vi "Pass.vi"(0 "Other Array":dbl[](array[numeric]), 1 "Other Boolean Array":bool[](array[boolean]), 2 "Denge Kosulu x2_y2":dbl[][](array[numeric]), 3 "LstBox Refnum":refnum<vi>, 4 "Cluster":T2, 5 "F/P Array Cluster":T1, 6 "Sheet name":string="10k1k", 7 "default values":T3(array[cluster]) {"Kelvin Yk-1" format="%.4p"; "Wagner Yk-1" format="%.4p"; "1R Yk-1" format="%.4p"; "10R Yk-1" format="%.4p"; "Ana Denge Yk-1" format="%.4p"; "Kelvin Yk" format="%.4p"; "Wagner Yk" format="%.4p"; "1R Yk" format="%.4p"; "10R Yk" format="%.4p"; "Ana Denge Yk" format="%.4p"; "Kelvin Xk-1" format="%.4p"; "Wagner Xk-1" format="%.4p"; "1R Xk-1" format="%.4p"; "10R Xk-1" format="%.4p"; "Ana Denge Xk-1" format="%.4p"; "Kelvin Xk" format="%.4p"; "Wagner Xk" format="%.4p"; "1R Xk" format="%.4p"; "10R Xk" format="%.4p"; "Ana Denge Xk" format="%.4p"}, 8 "x1_x2_y1_y2":dbl[][](array[numeric]), 9 "input values":dbl[](array[numeric])) -> (10 "new iterasyon Denge":dbl, 12 "output values":dbl[](array[numeric]), 13 "Output Other Boolean Array":bool[](array[boolean]), 14 "Output Cluster":T2, 15 "Output F/P Array Cluster":T1, 16 "output default values":T3(array[cluster]) {"Kelvin Yk-1" format="%.4p"; "Wagner Yk-1" format="%.4p"; "1R Yk-1" format="%.4p"; "10R Yk-1" format="%.4p"; "Ana Denge Yk-1" format="%.4p"; "Kelvin Yk" format="%.4p"; "Wagner Yk" format="%.4p"; "1R Yk" format="%.4p"; "10R Yk" format="%.4p"; "Ana Denge Yk" format="%.4p"; "Kelvin Xk-1" format="%.4p"; "Wagner Xk-1" format="%.4p"; "1R Xk-1" format="%.4p"; "10R Xk-1" format="%.4p"; "Ana Denge Xk-1" format="%.4p"; "Kelvin Xk" format="%.4p"; "Wagner Xk" format="%.4p"; "1R Xk" format="%.4p"; "10R Xk" format="%.4p"; "Ana Denge Xk" format="%.4p"}, 17 "Output Iterasyon Successful":dbl, 18 "Denge Seçimi":u8=4 min=1 max=5, 19 "end time":string)   [LabVIEW 2014]
uses:
  DB_Global_4_kart-Test.vi
  Sub_VI/show_sensitivity.vi
panel:
  in  "Kelvin F/P Array":dbl[][](array[numeric])
  in  "Wagner F/P Array":dbl[][](array[numeric])
  in  "1R F/P Array":dbl[][](array[numeric])
  in  "10R F/P Array":dbl[][](array[numeric])
  in  "AD F/P Array":dbl[][](array[numeric])
  in  "Frekanslar":dbl[](array[numeric])
  in  "F Values Array":dbl[][](array[numeric])
  in  "extra default values":dbl[][](array[numeric])
  in  "control hz array":dbl[][](array[numeric])
  in  "index r":dbl
  in  "iterasyon Denge":dbl
  in  "change switch":bool
  in  "denge degeri":dbl
  in  "reset values":bool
  in  "ölçüm":u16=3 min=1 max=100
  in  "set":u16=3 min=1 max=100
  in  "frekans index":dbl
  in  "RESET SENS Y":bool
  in  "Iterasyon Successful":dbl
  in  "RESET SENS X":bool
  in  "GPIB In":refnum<visa-resource-name>="GPIB0::8::INSTR"
  in  "pass hz":bool
  out "continue object":bool
  # "Denge Degeri\nIterasyon Successful\nindex r\nolcum\nset\nfrekans index\nIterasyon Denge"
  # "pass hz\nchange switch\nreset values\nreset sens x\nreset sens y"
  # "pass hz\nchange switch\nreset values\nreset sens x\nreset sens y"
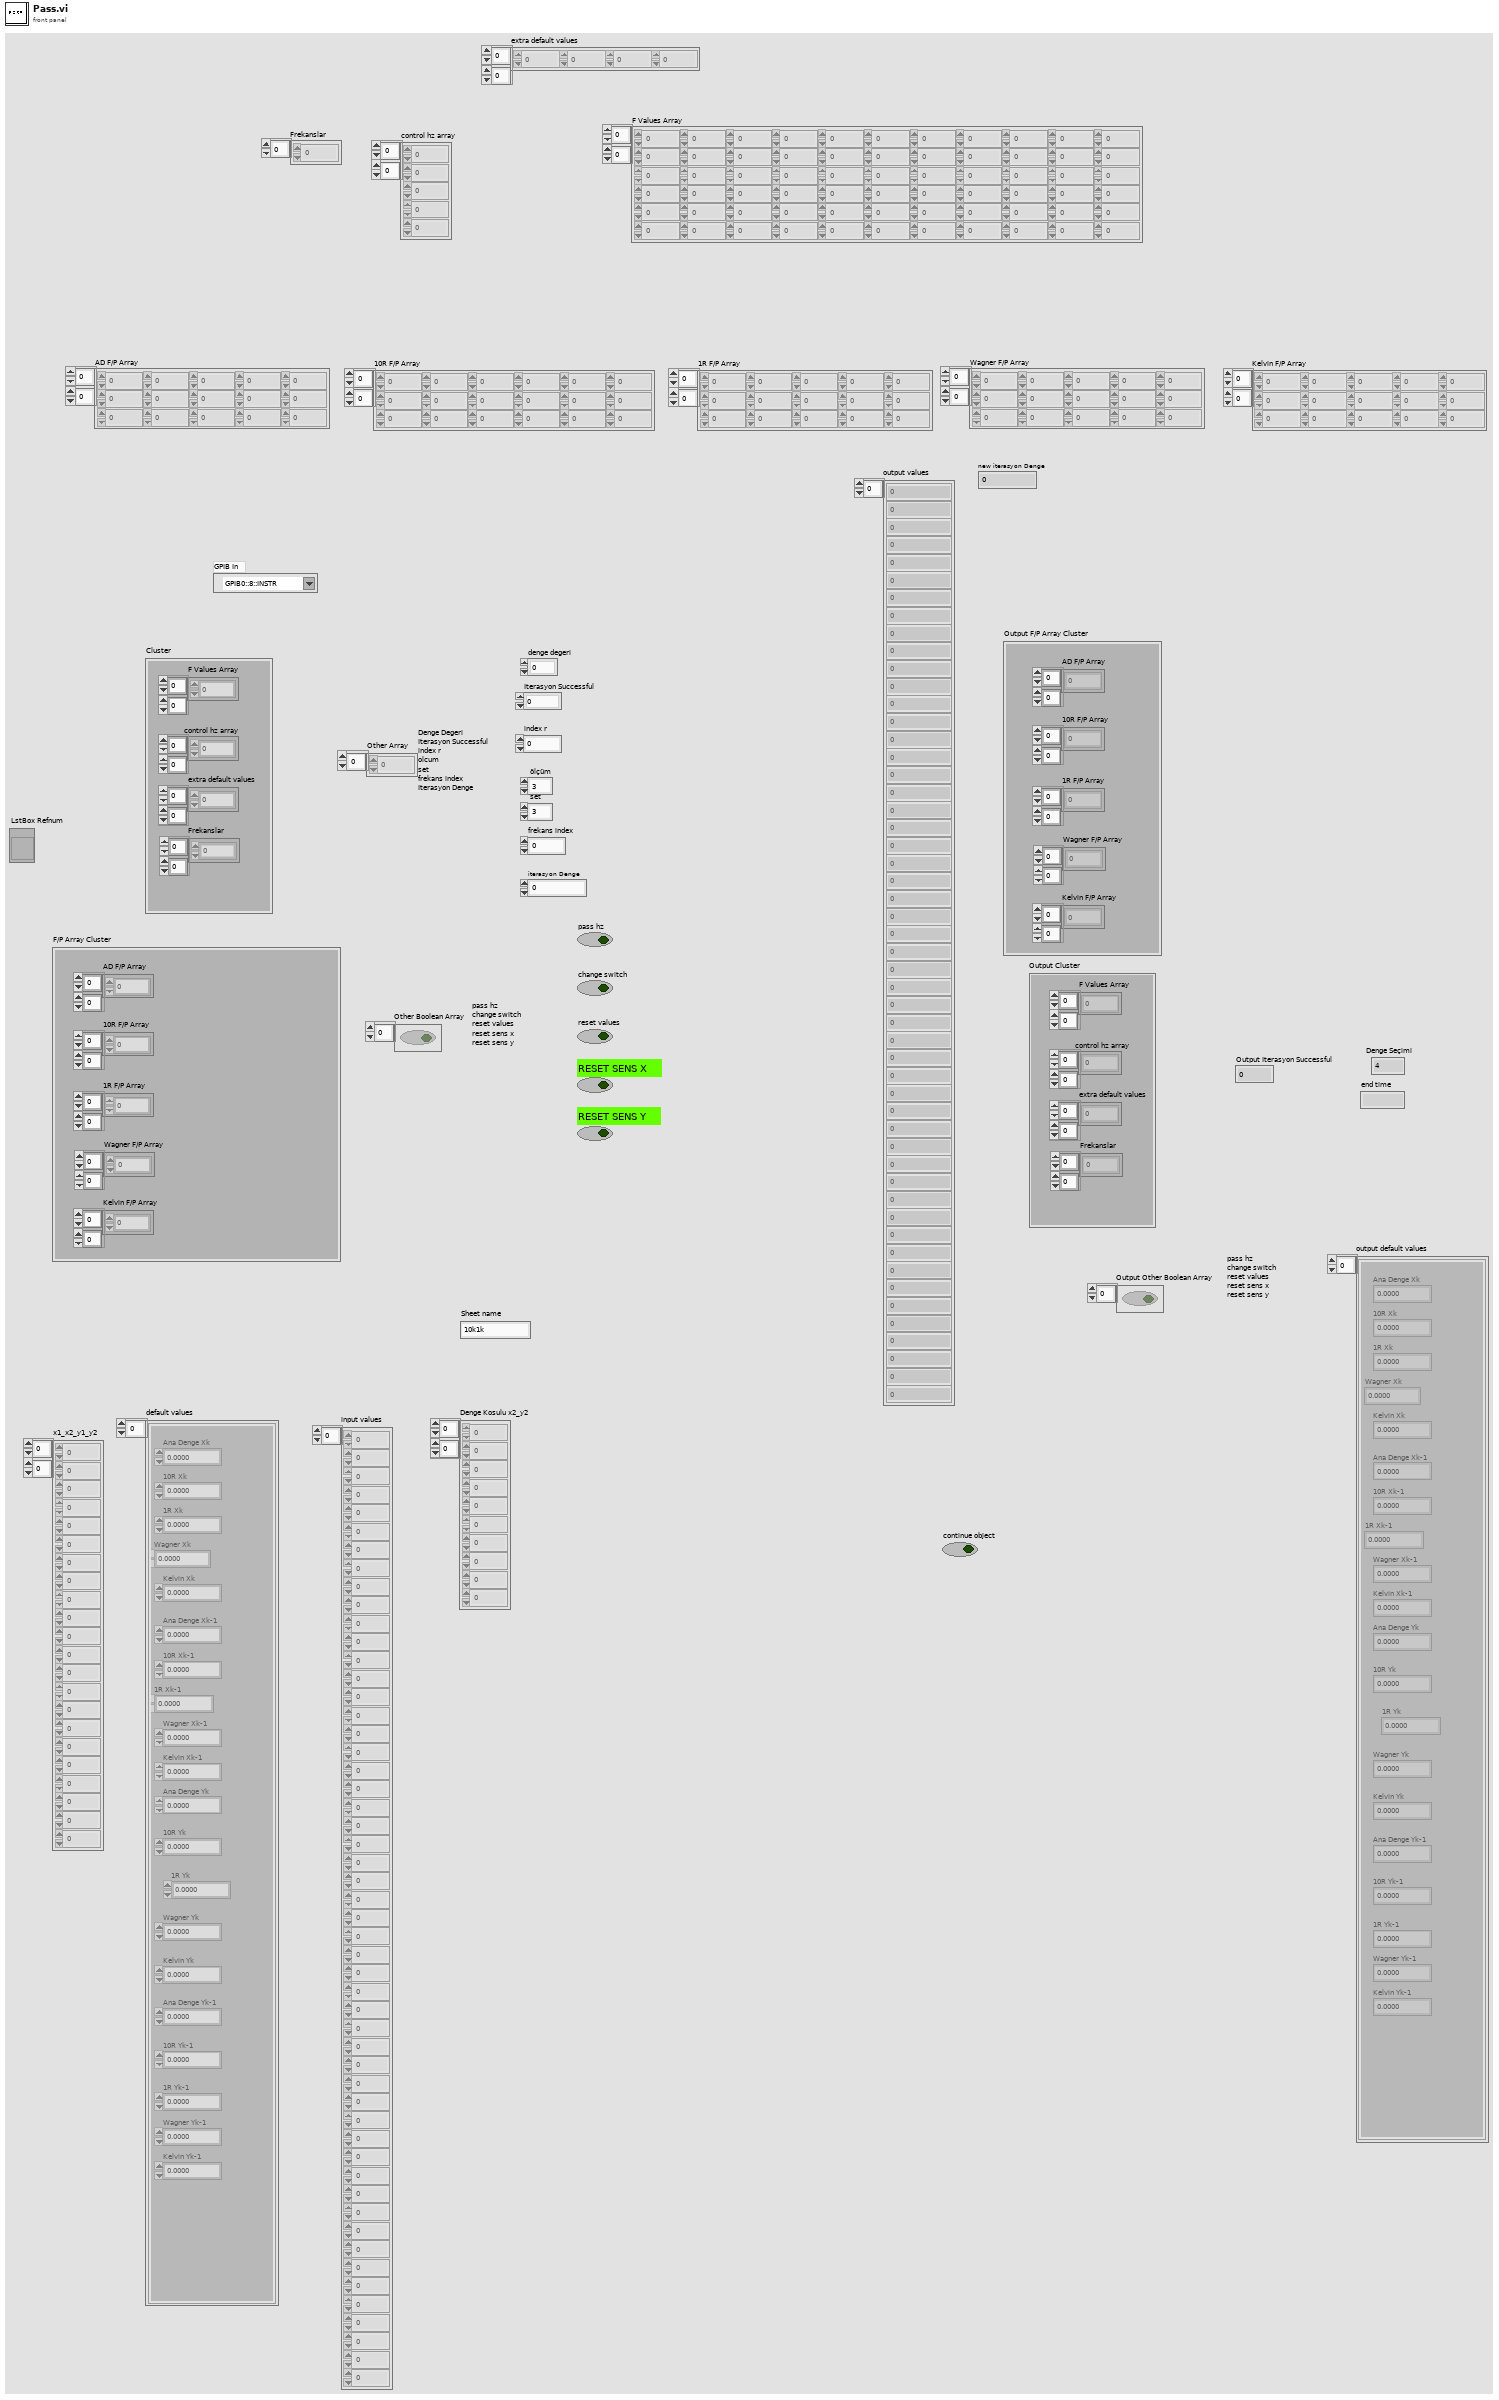
[diagram p1: front panel]
types:
  T1 = cluster{"AD F/P Array":dbl[][], "10R F/P Array":dbl[][], "1R F/P Array":dbl[][], "Wagner F/P Array":dbl[][], "Kelvin F/P Array":dbl[][]}
  T2 = cluster{"F Values Array":dbl[][], "control hz array":dbl[][], "extra default values":dbl[][], "Frekanslar":dbl[][]}
  T3 = cluster{"Ana Denge Xk":dbl, "10R Xk":dbl, "1R Xk":dbl, "Wagner Xk":dbl, "Kelvin Xk":dbl, "Ana Denge Xk-1":dbl, "10R Xk-1":dbl, "1R Xk-1":dbl, "Wagner Xk-1":dbl, "Kelvin Xk-1":dbl, "Ana Denge Yk":dbl, "10R Yk":dbl, "1R Yk":dbl, "Wagner Yk":dbl, "Kelvin Yk":dbl, "Ana Denge Yk-1":dbl, "10R Yk-1":dbl, "1R Yk-1":dbl, "Wagner Yk-1":dbl, "Kelvin Yk-1":dbl}[]
  T4 = cluster{"Ana Denge Xk":dbl, "10R Xk":dbl, "1R Xk":dbl, "Wagner Xk":dbl, "Kelvin Xk":dbl, "Ana Denge Xk-1":dbl, "10R Xk-1":dbl, "1R Xk-1":dbl, "Wagner Xk-1":dbl, "Kelvin Xk-1":dbl, "Ana Denge Yk":dbl, "10R Yk":dbl, "1R Yk":dbl, "Wagner Yk":dbl, "Kelvin Yk":dbl, "Ana Denge Yk-1":dbl, "10R Yk-1":dbl, "1R Yk-1":dbl, "Wagner Yk-1":dbl, "Kelvin Yk-1":dbl}
  T5 = cluster{"[0]":dbl, "[1]":dbl, "[2]":dbl, "[3]":dbl, "[4]":dbl, "[5]":dbl, "[6]":dbl, "[7]":dbl, "[8]":dbl, "[9]":dbl, "[10]":dbl, "[11]":dbl, "[12]":dbl, "[13]":dbl, "[14]":dbl, "[15]":dbl, "[16]":dbl, "[17]":dbl, "[18]":dbl, "[19]":dbl}
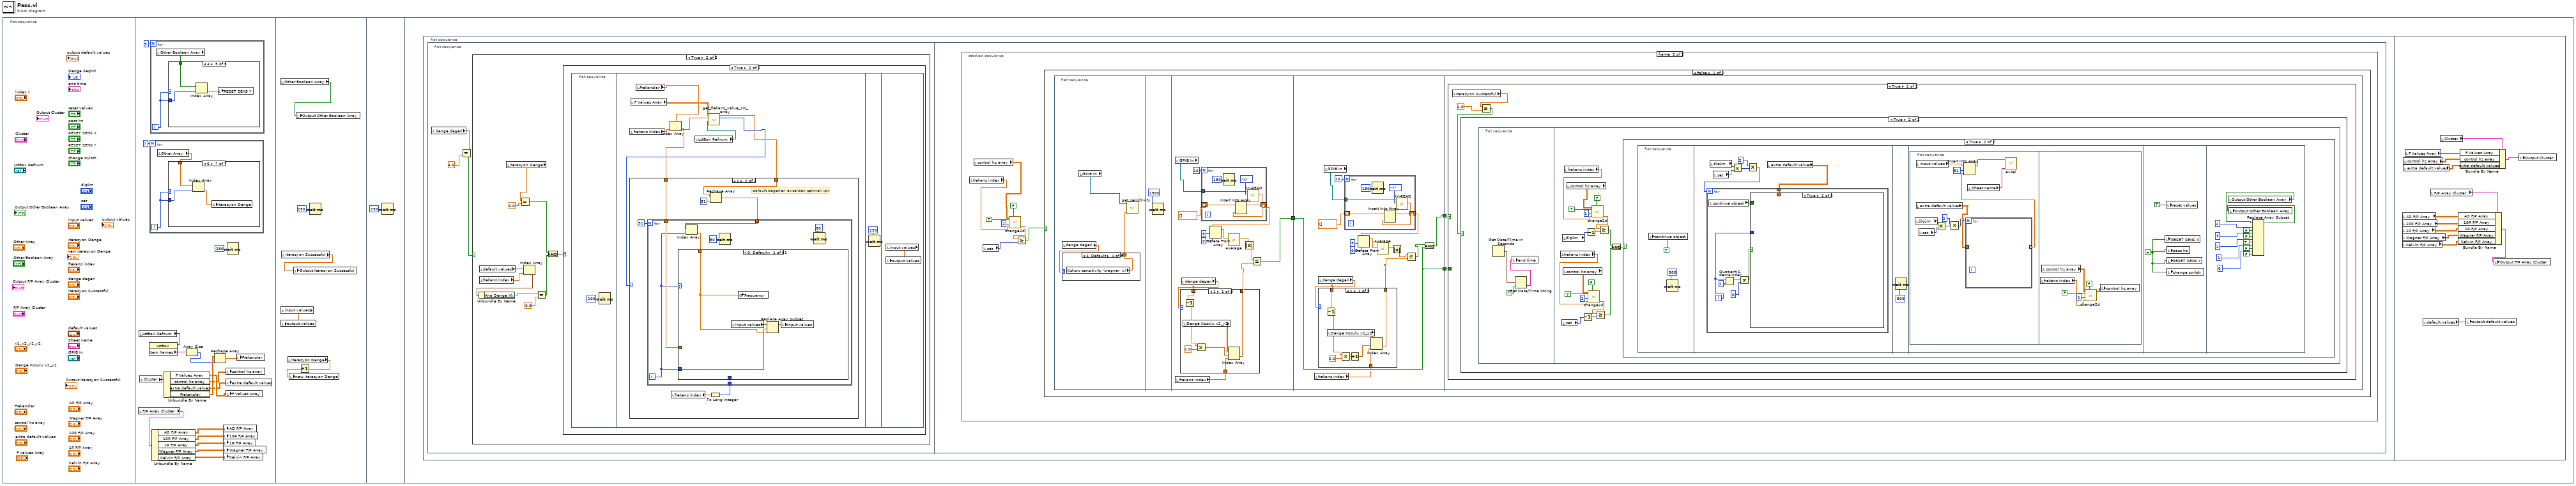
[diagram p0: block diagram]
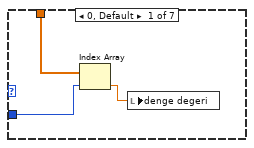
[diagram p2: hidden frame]
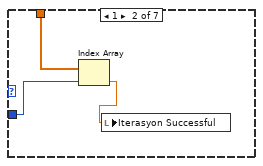
[diagram p3: hidden frame]
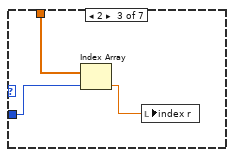
[diagram p4: hidden frame]
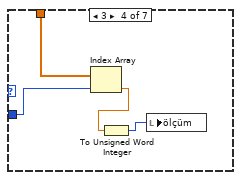
[diagram p5: hidden frame]
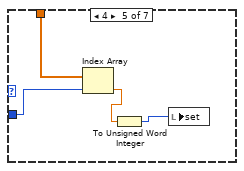
[diagram p6: hidden frame]
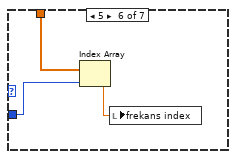
[diagram p7: hidden frame]
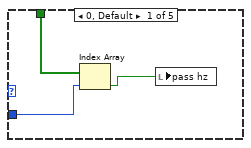
[diagram p8: hidden frame]
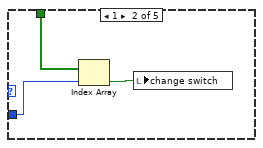
[diagram p9: hidden frame]
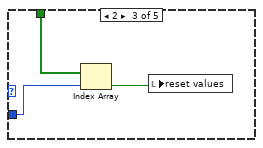
[diagram p10: hidden frame]
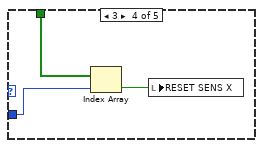
[diagram p11: hidden frame]
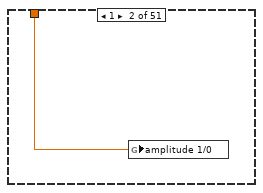
[diagram p15: hidden frame]
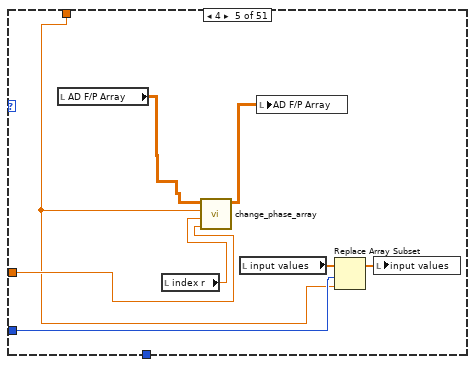
[diagram p18: hidden frame]
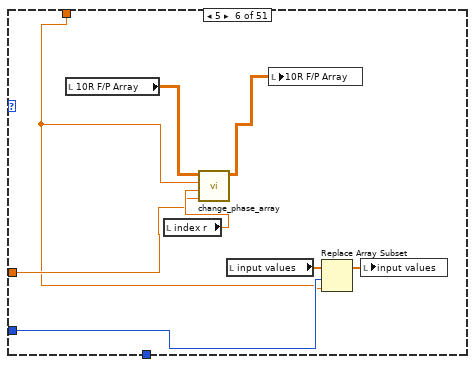
[diagram p19: hidden frame]
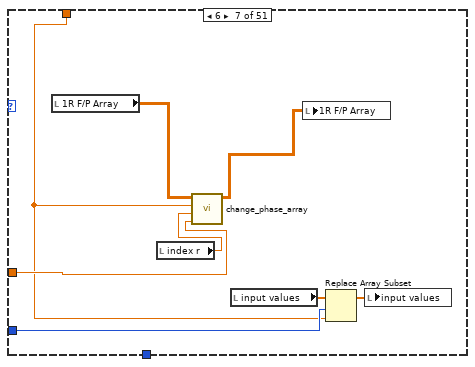
[diagram p20: hidden frame]
diagram:
  n1 = flat-sequence {
    frame #0 {
    }
    frame #1 {
      n2 = local read "F/P Array Cluster"() -> (w6:T1)
      n3 = local read "LstBox Refnum"() -> (w18:refnum<vi>)
      n4 = local read "Cluster"() -> (w12:T2)
      n5 = property class="LstBox"(reference=w18) -> ("Item Names"=w17:string[])  [unwired: 1 in, 2 out]
      n6 = for {
        N: 7 -> [_]
        i -> [w20]
        n7 = local read "Other Array"() -> (w19:dbl[])
        n8 = case shown="6" w20 {
          tunnel: w19 -> [w23 w26 w29 w33 w37 w40 w43]
          tunnel: w20 -> [w22 w25 w28 w32 w36 w39 w42]
          frame 0, Default {
            n9 = Index Array(array=w23, index=w22) -> (element=w21:dbl)
            n10 = local write "denge degeri"(w21) -> ()
          }
          frame 1 {
            n11 = Index Array(array=w26, index=w25) -> (element=w24:dbl)
            n12 = local write "Iterasyon Successful"(w24) -> ()
          }
          frame 2 {
            n13 = Index Array(array=w29, index=w28) -> (element=w27:dbl)
            n14 = local write "index r"(w27) -> ()
          }
          frame 3 {
            n15 = Index Array(array=w33, index=w32) -> (element=w31:dbl)
            n16 = To Unsigned Word Integer(number=w31) -> (unsigned 16bit integer=w30:u16)
            n17 = local write "ölçüm"(w30) -> ()
          }
          frame 4 {
            n18 = Index Array(array=w37, index=w36) -> (element=w34:dbl)
            n19 = To Unsigned Word Integer(number=w34) -> (unsigned 16bit integer=w35:u16)
            n20 = local write "set"(w35) -> ()
          }
          frame 5 {
            n21 = Index Array(array=w40, index=w39) -> (element=w38:dbl)
            n22 = local write "frekans index"(w38) -> ()
          }
          frame 6 {
            n23 = Index Array(array=w43, index=w42) -> (element=w41:dbl)
            n24 = local write "iterasyon Denge"(w41) -> ()
          }
        }
      }
      n25 = for {
        N: 5 -> [_]
        i -> [w44]
        n26 = local read "Other Boolean Array"() -> (w45:bool[])
        n27 = case shown="4" w44 {
          tunnel: w45 -> [w48 w51 w54 w57 w60]
          tunnel: w44 -> [w47 w50 w53 w56 w59]
          frame 0, Default {
            n28 = Index Array(array=w48, index=w47) -> (element=w46:bool)
            n29 = local write "pass hz"(w46) -> ()
          }
          frame 1 {
            n30 = Index Array(array=w51, index=w50) -> (element=w49:bool)
            n31 = local write "change switch"(w49) -> ()
          }
          frame 2 {
            n32 = Index Array(array=w54, index=w53) -> (element=w52:bool)
            n33 = local write "reset values"(w52) -> ()
          }
          frame 3 {
            n34 = Index Array(array=w57, index=w56) -> (element=w55:bool)
            n35 = local write "RESET SENS X"(w55) -> ()
          }
          frame 4 {
            n36 = Index Array(array=w60, index=w59) -> (element=w58:bool)
            n37 = local write "RESET SENS Y"(w58) -> ()
          }
        }
      }
      n38 = Unbundle By Name(w6) -> ("AD F/P Array"=w5:dbl[][], "10R F/P Array"=w4:dbl[][], "1R F/P Array"=w3:dbl[][], "Wagner F/P Array"=w2:dbl[][], "Kelvin F/P Array"=w1:dbl[][])
      n39 = Unbundle By Name(w12) -> ("F Values Array"=w10:dbl[][], "control hz array"=w8:dbl[][], "extra default values"=w9:dbl[][], "Frekanslar"=w11:dbl[][])
      n40 = Array Size(array=w17) -> (size(s)=w16:i32)
      n41 = Reshape Array(w11, w16) -> (w7:dbl[])
      n42 = local write "AD F/P Array"(w5) -> ()
      n43 = local write "10R F/P Array"(w4) -> ()
      n44 = local write "1R F/P Array"(w3) -> ()
      n45 = local write "Wagner F/P Array"(w2) -> ()
      n46 = local write "Kelvin F/P Array"(w1) -> ()
      n47 = local write "control hz array"(w8) -> ()
      n48 = local write "extra default values"(w9) -> ()
      n49 = local write "F Values Array"(w10) -> ()
      n50 = Wait (ms)(milliseconds to wait=u32 250) -> ()  [unwired: 1 out]
      n51 = local write "Frekanslar"(w7) -> ()
    }
    frame #2 {
      n52 = local read "Other Boolean Array"() -> (w65:bool[])
      n53 = local read "input values"() -> (w63:dbl[])
      n54 = local write "output values"(w63) -> ()
      n55 = local read "Iterasyon Successful"() -> (w66:dbl)
      n56 = local read "iterasyon Denge"() -> (w61:dbl)
      n57 = local write "Output Iterasyon Successful"(w66) -> ()
      n58 = local write "Output Other Boolean Array"(w65) -> ()
      n59 = Increment(x=w61) -> (x+1=w62:dbl)
      n60 = local write "new iterasyon Denge"(w62) -> ()
      n61 = Wait (ms)(milliseconds to wait=u32 250) -> ()  [unwired: 1 out]
    }
    frame #3 {
      n62 = Wait (ms)(milliseconds to wait=u32 250) -> ()  [unwired: 1 out]
    }
    frame #4 {
      n63 = flat-sequence {
        frame #0 {
          n64 = flat-sequence {
            frame #0 {
              n65 = local read "denge degeri"() -> (w69:dbl)
              n66 = Equal?(x=w69, y=4.0) -> (x = y?=w68:bool)
              n67 = case shown="True" w68 {
                frame False {
                }
                frame True {
                  n68 = local read "default values"() -> (w75:T3)
                  n69 = local read "frekans index"() -> (w74:dbl)
                  n70 = local read "iterasyon Denge"() -> (w72:dbl)
                  n71 = Equal?(x=w72, y=0.0) -> (x = y?=w78:bool)
                  n72 = Index Array(array=w75, index=w74) -> (element=w73:T4)
                  n73 = Unbundle By Name(w73) -> ("Ana Denge Xk"=w77:dbl)
                  n74 = Equal?(x=w77, y=0.0) -> (x = y?=w79:bool)
                  n75 = And(x=w78, y=w79) -> (x .and. y?=w80:bool)
                  n76 = case shown="True" w80 {
                    frame False {
                    }
                    frame True {
                      n77 = flat-sequence {
                        frame #0 {
                          n78 = Wait (ms)(milliseconds to wait=u32 100) -> ()  [unwired: 1 out]
                        }
                        frame #1 {
                          n79 = local read "frekans index"() -> (w88:dbl)
                          n80 = local read "F Values Array"() -> (w82:dbl[][])
                          n81 = local read "Frekanslar"() -> (w83:dbl[])
                          n82 = Index Array(array=w83, index=w88) -> (element=w85:dbl)
                          n83 = local read "LstBox Refnum"() -> (w84:refnum<vi>)
                          n84 = call "get_frekans_value_1D_array.vi"("LstBox Refnum"=w84, "frekans"=w85, "F Values Array"=w82) -> ("symbol enable?"=w87:i32, "output array"=w86:dbl[])  [unwired: 7 in]
                          n85 = case shown="1" w87 {
                            tunnel: w86 -> [_ w93]
                            tunnel: w85 -> [_ w92]
                            frame 10, Default {
                            }
                            frame 1 {
                              # "dafault değerleri excelden çekmek için"
                              n86 = local read "frekans index"() -> (w90:dbl)
                              n87 = To Long Integer(number=w90) -> (32bit integer=w89:i32)
                              n88 = Reshape Array(w93, 51 ("dimension size")) -> (w91:dbl[])
                              n89 = for {
                                N: 51 -> [_]
                                tunnel: w91 -> [w101]
                                tunnel: w92 -> [w99]
                                tunnel: w89 -> [w96]
                                i -> [w98]
                                n90 = Index Array(array=w101, index=w98) -> (element=w100:dbl)
                                n91 = case shown="0, Default" w98 {
                                tunnel: w100 -> [w103 w107 _ _ w108 w116 w124 w133 w145 w153 w157 w162 w165 w170 w173 w177 w181 w186 w189 w194 w198 w202 w205 w210 w213 w218 w221 w225 w230 _ _ _ _ _ _ _ _ _ _ _ _ _ _ _ _ _ _ _ _ _ _]
                                tunnel: w99 -> [_ _ _ _ w114 w122 w130 w143 w151 _ _ _ _ _ _ _ _ _ _ _ _ _ _ _ _ _ _ _ _ _ _ _ _ _ _ _ _ _ _ _ _ _ _ _ _ _ _ _ _ _ _]
                                tunnel: w98 -> [w104 _ _ _ w111 w119 w127 w140 w148 w154 w158 w161 w166 w169 w174 w178 w182 w185 w190 w193 w197 w201 w206 w209 w214 w217 w222 w226 w229 w234 w242 w250 w258 w266 w274 w282 w290 w298 w306 w314 w322 w330 w338 w346 w354 w362 w370 w378 w386 w398 w406]
                                tunnel: w96 -> [_ _ _ _ _ _ _ _ _ _ _ _ _ _ _ _ _ _ _ _ _ _ _ _ _ _ _ _ _ w233 w241 w249 w257 w265 w273 w281 w289 w297 w305 w313 w321 w329 w337 w345 w353 w361 w369 w377 w385 _ _]
                                frame 0, Default {
                                n92 = local read "input values"() -> (w105:dbl[])
                                n93 = global write "DB_Global_4_kart-Test.vi" "Frequency"(w103) -> ()
                                n94 = Replace Array Subset(array=w105, new element=w103, index=w104) -> (w106:dbl[])
                                n95 = local write "input values"(w106) -> ()
                                }
                                frame 1 {
                                n96 = global write "DB_Global_4_kart-Test.vi" "amplitude 1/0"(w107) -> ()
                                }
                                frame 2 {
                                }
                                frame 3 {
                                }
                                frame 4 {
                                n97 = local read "AD F/P Array"() -> (w110:dbl[][])
                                n98 = local read "index r"() -> (w115:dbl)
                                n99 = call "change_phase_array.vi"("frekans"=w114, "index r"=w115, "Change Phase"=w108, "Base Array"=w110) -> ("output array"=w109:dbl[][])  [unwired: 7 in]
                                n100 = local read "input values"() -> (w112:dbl[])
                                n101 = local write "AD F/P Array"(w109) -> ()
                                n102 = Replace Array Subset(array=w112, new element=w108, index=w111) -> (w113:dbl[])
                                n103 = local write "input values"(w113) -> ()
                                }
                                frame 5 {
                                n104 = local read "10R F/P Array"() -> (w118:dbl[][])
                                n105 = local read "index r"() -> (w123:dbl)
                                n106 = call "change_phase_array.vi"("frekans"=w122, "index r"=w123, "Change Phase"=w116, "Base Array"=w118) -> ("output array"=w117:dbl[][])  [unwired: 7 in]
                                n107 = local read "input values"() -> (w120:dbl[])
                                n108 = local write "10R F/P Array"(w117) -> ()
                                n109 = Replace Array Subset(array=w120, new element=w116, index=w119) -> (w121:dbl[])
                                n110 = local write "input values"(w121) -> ()
                                }
                                frame 6 {
                                n111 = local read "1R F/P Array"() -> (w126:dbl[][])
                                n112 = local read "index r"() -> (w131:dbl)
                                n113 = call "change_phase_array.vi"("frekans"=w130, "index r"=w131, "Change Phase"=w124, "Base Array"=w126) -> ("output array"=w125:dbl[][])  [unwired: 7 in]
                                n114 = local read "input values"() -> (w128:dbl[])
                                n115 = local write "1R F/P Array"(w125) -> ()
                                n116 = Replace Array Subset(array=w128, new element=w124, index=w127) -> (w129:dbl[])
                                n117 = local write "input values"(w129) -> ()
                                }
                                frame 7 {
                                n118 = local read "index r"() -> (w144:dbl)
                                n119 = Number To Fractional String(number=w133) -> (F-format string=w135:string)  [unwired: 3 in]
                                n120 = Search and Replace String(input string=w135, search string=",", replace string="." ("replace string (\"\")")) -> (result string=w137:string)  [unwired: 5 in, 3 out]
                                n121 = local read "GPIB In"() -> (w134:refnum<visa-resource-name>)
                                n122 = local read "Wagner F/P Array"() -> (w139:dbl[][])
                                n123 = call "reference phase.vi"("Reference Phase (0.000 degrees)"=w137, "VISA resource name"=w134) -> ()  [unwired: 8 in, 2 out]
                                n124 = local read "input values"() -> (w141:dbl[])
                                n125 = call "change_phase_array.vi"("frekans"=w143, "index r"=w144, "Change Phase"=w133, "Base Array"=w139) -> ("output array"=w138:dbl[][])  [unwired: 7 in]
                                n126 = local write "Wagner F/P Array"(w138) -> ()
                                n127 = Replace Array Subset(array=w141, new element=w133, index=w140) -> (w142:dbl[])
                                n128 = local write "input values"(w142) -> ()
                                }
                                frame 8 {
                                n129 = local read "Kelvin F/P Array"() -> (w147:dbl[][])
                                n130 = local read "index r"() -> (w152:dbl)
                                n131 = call "change_phase_array.vi"("frekans"=w151, "index r"=w152, "Change Phase"=w145, "Base Array"=w147) -> ("output array"=w146:dbl[][])  [unwired: 7 in]
                                n132 = local read "input values"() -> (w149:dbl[])
                                n133 = local write "Kelvin F/P Array"(w146) -> ()
                                n134 = Replace Array Subset(array=w149, new element=w145, index=w148) -> (w150:dbl[])
                                n135 = local write "input values"(w150) -> ()
                                }
                                frame 9 {
                                n136 = global write "DB_Global_4_kart-Test.vi" "amplitude 2/0"(w153) -> ()
                                n137 = local read "input values"() -> (w155:dbl[])
                                n138 = Replace Array Subset(array=w155, new element=w153, index=w154) -> (w156:dbl[])
                                n139 = local write "input values"(w156) -> ()
                                }
                                frame 10 {
                                n140 = global write "DB_Global_4_kart-Test.vi" "amplitude 3/0"(w157) -> ()
                                n141 = local read "input values"() -> (w159:dbl[])
                                n142 = Replace Array Subset(array=w159, new element=w157, index=w158) -> (w160:dbl[])
                                n143 = local write "input values"(w160) -> ()
                                }
                                frame 11 {
                                n144 = global write "DB_Global_4_kart-Test.vi" "amplitude 3/1"(w162) -> ()
                                n145 = local read "input values"() -> (w163:dbl[])
                                n146 = Replace Array Subset(array=w163, new element=w162, index=w161) -> (w164:dbl[])
                                n147 = local write "input values"(w164) -> ()
                                }
                                frame 12 {
                                n148 = global write "DB_Global_4_kart-Test.vi" "amplitude 1/1"(w165) -> ()
                                n149 = local read "input values"() -> (w167:dbl[])
                                n150 = Replace Array Subset(array=w167, new element=w165, index=w166) -> (w168:dbl[])
                                n151 = local write "input values"(w168) -> ()
                                }
                                frame 13 {
                                n152 = global write "DB_Global_4_kart-Test.vi" "amplitude 2/1"(w170) -> ()
                                n153 = local read "input values"() -> (w171:dbl[])
                                n154 = Replace Array Subset(array=w171, new element=w170, index=w169) -> (w172:dbl[])
                                n155 = local write "input values"(w172) -> ()
                                }
                                frame 14 {
                                n156 = local read "input values"() -> (w175:dbl[])
                                n157 = Replace Array Subset(array=w175, new element=w173, index=w174) -> (w176:dbl[])
                                n158 = local write "input values"(w176) -> ()
                                }
                                frame 15 {
                                n159 = local read "input values"() -> (w179:dbl[])
                                n160 = Replace Array Subset(array=w179, new element=w177, index=w178) -> (w180:dbl[])
                                n161 = local write "input values"(w180) -> ()
                                }
                                frame 16 {
                                n162 = local read "input values"() -> (w183:dbl[])
                                n163 = Replace Array Subset(array=w183, new element=w181, index=w182) -> (w184:dbl[])
                                n164 = local write "input values"(w184) -> ()
                                }
                                frame 17 {
                                n165 = local read "input values"() -> (w187:dbl[])
                                n166 = Replace Array Subset(array=w187, new element=w186, index=w185) -> (w188:dbl[])
                                n167 = local write "input values"(w188) -> ()
                                }
                                frame 18 {
                                n168 = local read "input values"() -> (w191:dbl[])
                                n169 = Replace Array Subset(array=w191, new element=w189, index=w190) -> (w192:dbl[])
                                n170 = local write "input values"(w192) -> ()
                                }
                                frame 19 {
                                n171 = global write "DB_Global_4_kart-Test.vi" "phase 2/ 0"(w194) -> ()
                                n172 = local read "input values"() -> (w195:dbl[])
                                n173 = Replace Array Subset(array=w195, new element=w194, index=w193) -> (w196:dbl[])
                                n174 = local write "input values"(w196) -> ()
                                }
                                frame 20 {
                                n175 = global write "DB_Global_4_kart-Test.vi" "phase 3/0"(w198) -> ()
                                n176 = local read "input values"() -> (w199:dbl[])
                                n177 = Replace Array Subset(array=w199, new element=w198, index=w197) -> (w200:dbl[])
                                n178 = local write "input values"(w200) -> ()
                                }
                                frame 21 {
                                n179 = global write "DB_Global_4_kart-Test.vi" "phase 3/1"(w202) -> ()
                                n180 = local read "input values"() -> (w203:dbl[])
                                n181 = Replace Array Subset(array=w203, new element=w202, index=w201) -> (w204:dbl[])
                                n182 = local write "input values"(w204) -> ()
                                }
                                frame 22 {
                                n183 = global write "DB_Global_4_kart-Test.vi" "phase 1/1"(w205) -> ()
                                n184 = local read "input values"() -> (w207:dbl[])
                                n185 = Replace Array Subset(array=w207, new element=w205, index=w206) -> (w208:dbl[])
                                n186 = local write "input values"(w208) -> ()
                                }
                                frame 23 {
                                n187 = global write "DB_Global_4_kart-Test.vi" "phase 2/1"(w210) -> ()
                                n188 = local read "input values"() -> (w211:dbl[])
                                n189 = Replace Array Subset(array=w211, new element=w210, index=w209) -> (w212:dbl[])
                                n190 = local write "input values"(w212) -> ()
                                }
                                frame 24 {
                                n191 = local read "input values"() -> (w215:dbl[])
                                n192 = Replace Array Subset(array=w215, new element=w213, index=w214) -> (w216:dbl[])
                                n193 = local write "input values"(w216) -> ()
                                }
                                frame 25 {
                                n194 = local read "input values"() -> (w219:dbl[])
                                n195 = Replace Array Subset(array=w219, new element=w218, index=w217) -> (w220:dbl[])
                                n196 = local write "input values"(w220) -> ()
                                }
                                frame 26 {
                                n197 = local read "input values"() -> (w223:dbl[])
                                n198 = Replace Array Subset(array=w223, new element=w221, index=w222) -> (w224:dbl[])
                                n199 = local write "input values"(w224) -> ()
                                }
                                frame 27 {
                                n200 = local read "input values"() -> (w227:dbl[])
                                n201 = Replace Array Subset(array=w227, new element=w225, index=w226) -> (w228:dbl[])
                                n202 = local write "input values"(w228) -> ()
                                }
                                frame 28 {
                                n203 = local read "input values"() -> (w231:dbl[])
                                n204 = Replace Array Subset(array=w231, new element=w230, index=w229) -> (w232:dbl[])
                                n205 = local write "input values"(w232) -> ()
                                }
                                frame 29 {
                                n206 = local read "x1_x2_y1_y2"() -> (w238:dbl[][])
                                n207 = Subtract(x=w234, y=29 ("x")) -> (x-y=w237:i32)
                                n208 = Index Array(array=w238, index (row)=w237, index (col)=w233) -> (element=w236:dbl)
                                n209 = local read "input values"() -> (w239:dbl[])
                                n210 = Replace Array Subset(array=w239, new element=w236, index=w234) -> (w240:dbl[])
                                n211 = local write "input values"(w240) -> ()
                                }
                                frame 30 {
                                n212 = local read "x1_x2_y1_y2"() -> (w246:dbl[][])
                                n213 = Subtract(x=w242, y=29 ("x")) -> (x-y=w245:i32)
                                n214 = Index Array(array=w246, index (row)=w245, index (col)=w241) -> (element=w244:dbl)
                                n215 = local read "input values"() -> (w247:dbl[])
                                n216 = Replace Array Subset(array=w247, new element=w244, index=w242) -> (w248:dbl[])
                                n217 = local write "input values"(w248) -> ()
                                }
                                frame 31 {
                                n218 = local read "x1_x2_y1_y2"() -> (w254:dbl[][])
                                n219 = Subtract(x=w250, y=29 ("x")) -> (x-y=w253:i32)
                                n220 = Index Array(array=w254, index (row)=w253, index (col)=w249) -> (element=w252:dbl)
                                n221 = local read "input values"() -> (w255:dbl[])
                                n222 = Replace Array Subset(array=w255, new element=w252, index=w250) -> (w256:dbl[])
                                n223 = local write "input values"(w256) -> ()
                                }
                                frame 32 {
                                n224 = local read "x1_x2_y1_y2"() -> (w262:dbl[][])
                                n225 = Subtract(x=w258, y=29 ("x")) -> (x-y=w261:i32)
                                n226 = Index Array(array=w262, index (row)=w261, index (col)=w257) -> (element=w260:dbl)
                                n227 = local read "input values"() -> (w263:dbl[])
                                n228 = Replace Array Subset(array=w263, new element=w260, index=w258) -> (w264:dbl[])
                                n229 = local write "input values"(w264) -> ()
                                }
                                frame 33 {
                                n230 = local read "x1_x2_y1_y2"() -> (w270:dbl[][])
                                n231 = Subtract(x=w266, y=29 ("x")) -> (x-y=w269:i32)
                                n232 = Index Array(array=w270, index (row)=w269, index (col)=w265) -> (element=w268:dbl)
                                n233 = local read "input values"() -> (w271:dbl[])
                                n234 = Replace Array Subset(array=w271, new element=w268, index=w266) -> (w272:dbl[])
                                n235 = local write "input values"(w272) -> ()
                                }
                                frame 34 {
                                n236 = local read "x1_x2_y1_y2"() -> (w278:dbl[][])
                                n237 = Subtract(x=w274, y=29 ("x")) -> (x-y=w277:i32)
                                n238 = Index Array(array=w278, index (row)=w277, index (col)=w273) -> (element=w276:dbl)
                                n239 = local read "input values"() -> (w279:dbl[])
                                n240 = Replace Array Subset(array=w279, new element=w276, index=w274) -> (w280:dbl[])
                                n241 = local write "input values"(w280) -> ()
                                }
                                frame 35 {
                                n242 = local read "x1_x2_y1_y2"() -> (w286:dbl[][])
                                n243 = Subtract(x=w282, y=29 ("x")) -> (x-y=w285:i32)
                                n244 = Index Array(array=w286, index (row)=w285, index (col)=w281) -> (element=w284:dbl)
                                n245 = local read "input values"() -> (w287:dbl[])
                                n246 = Replace Array Subset(array=w287, new element=w284, index=w282) -> (w288:dbl[])
                                n247 = local write "input values"(w288) -> ()
                                }
                                frame 36 {
                                n248 = local read "x1_x2_y1_y2"() -> (w294:dbl[][])
                                n249 = Subtract(x=w290, y=29 ("x")) -> (x-y=w293:i32)
                                n250 = Index Array(array=w294, index (row)=w293, index (col)=w289) -> (element=w292:dbl)
                                n251 = local read "input values"() -> (w295:dbl[])
                                n252 = Replace Array Subset(array=w295, new element=w292, index=w290) -> (w296:dbl[])
                                n253 = local write "input values"(w296) -> ()
                                }
                                frame 37 {
                                n254 = local read "x1_x2_y1_y2"() -> (w302:dbl[][])
                                n255 = Subtract(x=w298, y=29 ("x")) -> (x-y=w301:i32)
                                n256 = Index Array(array=w302, index (row)=w301, index (col)=w297) -> (element=w300:dbl)
                                n257 = local read "input values"() -> (w303:dbl[])
                                n258 = Replace Array Subset(array=w303, new element=w300, index=w298) -> (w304:dbl[])
                                n259 = local write "input values"(w304) -> ()
                                }
                                frame 38 {
                                n260 = local read "x1_x2_y1_y2"() -> (w310:dbl[][])
                                n261 = Subtract(x=w306, y=29 ("x")) -> (x-y=w309:i32)
                                n262 = Index Array(array=w310, index (row)=w309, index (col)=w305) -> (element=w308:dbl)
                                n263 = local read "input values"() -> (w311:dbl[])
                                n264 = Replace Array Subset(array=w311, new element=w308, index=w306) -> (w312:dbl[])
                                n265 = local write "input values"(w312) -> ()
                                }
                                frame 39 {
                                n266 = local read "x1_x2_y1_y2"() -> (w318:dbl[][])
                                n267 = Subtract(x=w314, y=29 ("x")) -> (x-y=w317:i32)
                                n268 = Index Array(array=w318, index (row)=w317, index (col)=w313) -> (element=w316:dbl)
                                n269 = local read "input values"() -> (w319:dbl[])
                                n270 = Replace Array Subset(array=w319, new element=w316, index=w314) -> (w320:dbl[])
                                n271 = local write "input values"(w320) -> ()
                                }
                                frame 40 {
                                n272 = local read "x1_x2_y1_y2"() -> (w326:dbl[][])
                                n273 = Subtract(x=w322, y=29 ("x")) -> (x-y=w325:i32)
                                n274 = Index Array(array=w326, index (row)=w325, index (col)=w321) -> (element=w324:dbl)
                                n275 = local read "input values"() -> (w327:dbl[])
                                n276 = Replace Array Subset(array=w327, new element=w324, index=w322) -> (w328:dbl[])
                                n277 = local write "input values"(w328) -> ()
                                }
                                frame 41 {
                                n278 = local read "x1_x2_y1_y2"() -> (w334:dbl[][])
                                n279 = Subtract(x=w330, y=29 ("x")) -> (x-y=w333:i32)
                                n280 = Index Array(array=w334, index (row)=w333, index (col)=w329) -> (element=w332:dbl)
                                n281 = local read "input values"() -> (w335:dbl[])
                                n282 = Replace Array Subset(array=w335, new element=w332, index=w330) -> (w336:dbl[])
                                n283 = local write "input values"(w336) -> ()
                                }
                                frame 42 {
                                n284 = local read "x1_x2_y1_y2"() -> (w342:dbl[][])
                                n285 = Subtract(x=w338, y=29 ("x")) -> (x-y=w341:i32)
                                n286 = Index Array(array=w342, index (row)=w341, index (col)=w337) -> (element=w340:dbl)
                                n287 = local read "input values"() -> (w343:dbl[])
                                n288 = Replace Array Subset(array=w343, new element=w340, index=w338) -> (w344:dbl[])
                                n289 = local write "input values"(w344) -> ()
                                }
                                frame 43 {
                                n290 = local read "x1_x2_y1_y2"() -> (w350:dbl[][])
                                n291 = Subtract(x=w346, y=29 ("x")) -> (x-y=w349:i32)
                                n292 = Index Array(array=w350, index (row)=w349, index (col)=w345) -> (element=w348:dbl)
                                n293 = local read "input values"() -> (w351:dbl[])
                                n294 = Replace Array Subset(array=w351, new element=w348, index=w346) -> (w352:dbl[])
                                n295 = local write "input values"(w352) -> ()
                                }
                                frame 44 {
                                n296 = local read "x1_x2_y1_y2"() -> (w358:dbl[][])
                                n297 = Subtract(x=w354, y=29 ("x")) -> (x-y=w357:i32)
                                n298 = Index Array(array=w358, index (row)=w357, index (col)=w353) -> (element=w356:dbl)
                                n299 = local read "input values"() -> (w359:dbl[])
                                n300 = Replace Array Subset(array=w359, new element=w356, index=w354) -> (w360:dbl[])
                                n301 = local write "input values"(w360) -> ()
                                }
                                frame 45 {
                                n302 = local read "x1_x2_y1_y2"() -> (w366:dbl[][])
                                n303 = Subtract(x=w362, y=29 ("x")) -> (x-y=w365:i32)
                                n304 = Index Array(array=w366, index (row)=w365, index (col)=w361) -> (element=w364:dbl)
                                n305 = local read "input values"() -> (w367:dbl[])
                                n306 = Replace Array Subset(array=w367, new element=w364, index=w362) -> (w368:dbl[])
                                n307 = local write "input values"(w368) -> ()
                                }
                                frame 46 {
                                n308 = local read "x1_x2_y1_y2"() -> (w374:dbl[][])
                                n309 = Subtract(x=w370, y=29 ("x")) -> (x-y=w373:i32)
                                n310 = Index Array(array=w374, index (row)=w373, index (col)=w369) -> (element=w372:dbl)
                                n311 = local read "input values"() -> (w375:dbl[])
                                n312 = Replace Array Subset(array=w375, new element=w372, index=w370) -> (w376:dbl[])
                                n313 = local write "input values"(w376) -> ()
                                }
                                frame 47 {
                                n314 = local read "x1_x2_y1_y2"() -> (w382:dbl[][])
                                n315 = Subtract(x=w378, y=29 ("x")) -> (x-y=w381:i32)
                                n316 = Index Array(array=w382, index (row)=w381, index (col)=w377) -> (element=w380:dbl)
                                n317 = local read "input values"() -> (w383:dbl[])
                                n318 = Replace Array Subset(array=w383, new element=w380, index=w378) -> (w384:dbl[])
                                n319 = local write "input values"(w384) -> ()
                                }
                                frame 48 {
                                n320 = local read "x1_x2_y1_y2"() -> (w390:dbl[][])
                                n321 = Subtract(x=w386, y=29 ("x")) -> (x-y=w389:i32)
                                n322 = Index Array(array=w390, index (row)=w389, index (col)=w385) -> (element=w388:dbl)
                                n323 = local read "input values"() -> (w391:dbl[])
                                n324 = Replace Array Subset(array=w391, new element=w388, index=w386) -> (w392:dbl[])
                                n325 = local write "input values"(w392) -> ()
                                }
                                frame 49 {
                                n326 = local read "F Values Array"() -> (w395:dbl[][])
                                n327 = local read "LstBox Refnum"() -> (w396:refnum<vi>)
                                n328 = local read "frekans index"() -> (w394:dbl)
                                n329 = local read "Frekanslar"() -> (w397:dbl[])
                                n330 = call "rlc.vi"("LstBox Refnum"=w396, "F values array"=w395, "Frekanslar"=w397, "frekans index"=w394) -> ("10R values"=w393:dbl)  [unwired: 14 in, 1 out]
                                n331 = local read "input values"() -> (w399:dbl[])
                                n332 = Replace Array Subset(array=w399, new element=w393, index=w398) -> (w400:dbl[])
                                n333 = local write "input values"(w400) -> ()
                                }
                                frame 50 {
                                n334 = local read "F Values Array"() -> (w404:dbl[][])
                                n335 = local read "LstBox Refnum"() -> (w405:refnum<vi>)
                                n336 = local read "frekans index"() -> (w403:dbl)
                                n337 = local read "Frekanslar"() -> (w402:dbl[])
                                n338 = call "rlc.vi"("LstBox Refnum"=w405, "F values array"=w404, "Frekanslar"=w402, "frekans index"=w403) -> ("1R values"=w401:dbl)  [unwired: 14 in, 1 out]
                                n339 = local read "input values"() -> (w407:dbl[])
                                n340 = Replace Array Subset(array=w407, new element=w401, index=w406) -> (w408:dbl[])
                                n341 = local write "input values"(w408) -> ()
                                }
                                }
                                n342 = Wait (ms)(milliseconds to wait=u32 50) -> ()  [unwired: 1 out]
                                n343 = Wait (ms)(milliseconds to wait=u32 50) -> ()  [unwired: 1 out]
                              }
                            }
                          }
                        }
                        frame #2 {
                          n344 = Wait (ms)(milliseconds to wait=u32 250) -> ()  [unwired: 1 out]
                        }
                        frame #3 {
                          n345 = local read "input values"() -> (w410:dbl[])
                          n346 = local write "output values"(w410) -> ()
                        }
                      }
                    }
                  }
                }
              }
            }
            frame #1 {
              n347 = stacked-sequence {
                frame #0 {
                }
                frame #1 {
                  n348 = local read "frekans index"() -> (w418:dbl)
                  n349 = local read "control hz array"() -> (w412:dbl[][])
                  n350 = local read "set"() -> (w414:u16)
                  n351 = call "change2d.vi"("reset(default false)"=FALSE, "index (col)"=w418, "index (row)"=2, "read/write(T/F)"=TRUE, "2D Array"=w412) -> ("result count"=w417:dbl)  [unwired: 5 in, 1 out]
                  n352 = Greater Or Equal?(x=w417, y=w414) -> (x >= y?=w411:bool)
                  n353 = case shown="False" w411 {
                    frame False {
                      n354 = flat-sequence {
                        tunnel: [w435] -> w421
                        tunnel: w421 -> [w488]
                        tunnel: [w489] -> w420
                        tunnel: [w488] -> w419
                        tunnel: w420 -> [w547]
                        tunnel: w419 -> [w546]
                        frame #0 {
                          n355 = local read "denge degeri"() -> (w423:dbl)
                          n356 = case shown="4, Default" w423 {
                            tunnel: [w425 w426 w427 w428 w429] -> w422
                            frame 1 {
                              n357 = global read "show_sensitivity.vi" "show sensitivity (ana denge  x)"() -> (w425:dbl)
                            }
                            frame 2 {
                              n358 = global read "show_sensitivity.vi" "show sensitivity (10R  x)"() -> (w426:dbl)
                            }
                            frame 3 {
                              n359 = global read "show_sensitivity.vi" "show sensitivity (1R  x)"() -> (w427:dbl)
                            }
                            frame 4, Default {
                              n360 = global read "show_sensitivity.vi" "show sensitivity (wagner  x)"() -> (w428:dbl)
                            }
                            frame 5 {
                              n361 = global read "show_sensitivity.vi" "show sensitivity (kelvin  x)"() -> (w429:dbl)
                            }
                          }
                          n362 = local read "GPIB In"() -> (w424:refnum<visa-resource-name>)
                          n363 = call "get_sensitivity.vi"("input 1"=w422, "SR850 GPIB In"=w424) -> ()  [unwired: 8 in, 2 out]
                        }
                        frame #1 {
                          n364 = Wait (ms)(milliseconds to wait=u32 1500) -> ()  [unwired: 1 out]
                        }
                        frame #2 {
                          n365 = local read "GPIB In"() -> (w437:refnum<visa-resource-name>)
                          n366 = local read "frekans index"() -> (w431:dbl)
                          n367 = local read "denge degeri"() -> (w432:dbl)
                          n368 = case shown="1" w432 {
                            tunnel: [w447 w454 w461 w468 w475] -> w433
                            tunnel: w432 -> [w448 w455 w462 w469 w476]
                            tunnel: w431 -> [w444 w451 w458 w465 w472]
                            frame 1 {
                              n369 = local read "Denge Kosulu x2_y2"() -> (w450:dbl[][])
                              n370 = Decrement(x=w448) -> (x-1=w446:dbl)
                              n371 = Multiply(x=w446, y=2.0) -> (x*y=w445:dbl)
                              n372 = Index Array(array=w450, index (row)=w445, index (col)=w444) -> (element=w447:dbl)
                            }
                            frame 2 {
                              n373 = Decrement(x=w455) -> (x-1=w453:dbl)
                              n374 = local read "Denge Kosulu x2_y2"() -> (w457:dbl[][])
                              n375 = Multiply(x=w453, y=2.0) -> (x*y=w452:dbl)
                              n376 = Index Array(array=w457, index (row)=w452, index (col)=w451) -> (element=w454:dbl)
                            }
                            frame 3 {
                              n377 = Decrement(x=w462) -> (x-1=w460:dbl)
                              n378 = local read "Denge Kosulu x2_y2"() -> (w464:dbl[][])
                              n379 = Multiply(x=w460, y=2.0) -> (x*y=w459:dbl)
                              n380 = Index Array(array=w464, index (row)=w459, index (col)=w458) -> (element=w461:dbl)
                            }
                            frame 4, Default {
                              n381 = Decrement(x=w469) -> (x-1=w467:dbl)
                              n382 = local read "Denge Kosulu x2_y2"() -> (w471:dbl[][])
                              n383 = Multiply(x=w467, y=2.0) -> (x*y=w466:dbl)
                              n384 = Index Array(array=w471, index (row)=w466, index (col)=w465) -> (element=w468:dbl)
                            }
                            frame 5 {
                              n385 = Decrement(x=w476) -> (x-1=w474:dbl)
                              n386 = local read "Denge Kosulu x2_y2"() -> (w478:dbl[][])
                              n387 = Multiply(x=w474, y=2.0) -> (x*y=w473:dbl)
                              n388 = Index Array(array=w478, index (row)=w473, index (col)=w472) -> (element=w475:dbl)
                            }
                          }
                          n389 = for {
                            N: 10 -> [_]
                            tunnel: w437 -> [w483]
                            shift-right: [w480] -> w440
                            shift-left: dbl[] [] -> [w481]
                            n390 = Wait (ms)(milliseconds to wait=u32 150) -> ()  [unwired: 1 out]
                            n391 = call "XY-READ.vi"("X/Y ?"=enum16{"X", "Y"}."X" ("Enum"), "SR850 GPIB IN"=w483) -> ("SR850_Reading"=w482:dbl)  [unwired: 7 in, 2 out]
                            n392 = Insert Into Array(array=w481, new element=w482) -> (w480:dbl[])  [unwired: 1 in]
                          }
                          n393 = Delete From Array(array=w440, length=5, index=0) -> (array with subset deleted=w441:dbl[])  [unwired: 1 out]
                          n394 = call "Average.vi"("Array"=w441) -> ("Average"=w436:dbl)  [unwired: 9 in, 1 out]
                          n395 = Absolute Value(x=w436) -> (abs(x)=w434:dbl)
                          n396 = Less Or Equal?(x=w434, y=w433) -> (x <= y?=w435:bool)
                        }
                        frame #3 {
                          n397 = local read "frekans index"() -> (w485:dbl)
                          n398 = local read "denge degeri"() -> (w486:dbl)
                          n399 = case shown="1" w486 {
                            tunnel: [w503 w511 w519 w527 w535] -> w487
                            tunnel: w486 -> [w504 w512 w520 w528 w536]
                            tunnel: w485 -> [w500 w508 w516 w524 w532]
                            frame 1 {
                              n400 = Decrement(x=w504) -> (x-1=w502:dbl)
                              n401 = local read "Denge Kosulu x2_y2"() -> (w506:dbl[][])
                              n402 = Multiply(x=w502, y=2.0) -> (x*y=w507:dbl)
                              n403 = Increment(x=w507) -> (x+1=w501:dbl)
                              n404 = Index Array(array=w506, index (row)=w501, index (col)=w500) -> (element=w503:dbl)
                            }
                            frame 2 {
                              n405 = Decrement(x=w512) -> (x-1=w510:dbl)
                              n406 = local read "Denge Kosulu x2_y2"() -> (w514:dbl[][])
                              n407 = Multiply(x=w510, y=2.0) -> (x*y=w515:dbl)
                              n408 = Increment(x=w515) -> (x+1=w509:dbl)
                              n409 = Index Array(array=w514, index (row)=w509, index (col)=w508) -> (element=w511:dbl)
                            }
                            frame 3 {
                              n410 = Decrement(x=w520) -> (x-1=w518:dbl)
                              n411 = local read "Denge Kosulu x2_y2"() -> (w522:dbl[][])
                              n412 = Multiply(x=w518, y=2.0) -> (x*y=w523:dbl)
                              n413 = Increment(x=w523) -> (x+1=w517:dbl)
                              n414 = Index Array(array=w522, index (row)=w517, index (col)=w516) -> (element=w519:dbl)
                            }
                            frame 4, Default {
                              n415 = Decrement(x=w528) -> (x-1=w526:dbl)
                              n416 = local read "Denge Kosulu x2_y2"() -> (w530:dbl[][])
                              n417 = Multiply(x=w526, y=2.0) -> (x*y=w531:dbl)
                              n418 = Increment(x=w531) -> (x+1=w525:dbl)
                              n419 = Index Array(array=w530, index (row)=w525, index (col)=w524) -> (element=w527:dbl)
                            }
                            frame 5 {
                              n420 = local read "Denge Kosulu x2_y2"() -> (w538:dbl[][])
                              n421 = Decrement(x=w536) -> (x-1=w534:dbl)
                              n422 = Multiply(x=w534, y=2.0) -> (x*y=w539:dbl)
                              n423 = Increment(x=w539) -> (x+1=w533:dbl)
                              n424 = Index Array(array=w538, index (row)=w533, index (col)=w532) -> (element=w535:dbl)
                            }
                          }
                          n425 = local read "GPIB In"() -> (w499:refnum<visa-resource-name>)
                          n426 = for {
                            N: 10 -> [_]
                            tunnel: w499 -> [w544]
                            shift-right: [w541] -> w496
                            shift-left: dbl[] [] -> [w542]
                            n427 = Wait (ms)(milliseconds to wait=u32 150) -> ()  [unwired: 1 out]
                            n428 = call "XY-READ.vi"("X/Y ?"=enum16{"X", "Y"}."Y" ("Enum"), "SR850 GPIB IN"=w544) -> ("SR850_Reading"=w543:dbl)  [unwired: 7 in, 2 out]
                            n429 = Insert Into Array(array=w542, new element=w543) -> (w541:dbl[])  [unwired: 1 in]
                          }
                          n430 = Delete From Array(array=w496, length=5, index=0) -> (array with subset deleted=w495:dbl[])  [unwired: 1 out]
                          n431 = call "Average.vi"("Array"=w495) -> ("Average"=w492:dbl)  [unwired: 9 in, 1 out]
                          n432 = Absolute Value(x=w492) -> (abs(x)=w491:dbl)
                          n433 = Less Or Equal?(x=w491, y=w487) -> (x <= y?=w490:bool)
                          n434 = And(x=w490, y=w488) -> (x .and. y?=w489:bool)
                        }
                        frame #4 {
                          n435 = case shown="True" w547 {
                            tunnel: w546 -> [w548 _]
                            frame False {
                              n436 = case shown="False" w548 {
                                frame False {
                                n437 = flat-sequence {
                                frame #0 {
                                w550 = FALSE ("START X")
                                n438 = local write "Output Iterasyon Successful"(0.0 ("Iterasyon Successful")) -> ()
                                n439 = local write "RESET SENS X"(TRUE ("RESET SENS X")) -> ()
                                n440 = local write "reset values"(w550) -> ()
                                n441 = local write "pass hz"(w550) -> ()
                                n442 = local write "RESET SENS Y"(w550) -> ()
                                n443 = local write "change switch"(w550) -> ()
                                }
                                frame #1 {
                                n444 = local read "Output Other Boolean Array"() -> (w562:bool[])
                                n445 = Replace Array Subset(array=w562, new element #1=FALSE ("new element/subarray"), index #1=4 ("index"), new element #2=TRUE ("new element/subarray"), index #2=3 ("index"), new element #3=FALSE ("new element/subarray"), index #3=2 ("index"), new element #4=FALSE ("new element/subarray"), index #4=1 ("index"), new element #5=FALSE ("new element/subarray"), index #5=0 ("index")) -> (w563:bool[])
                                n446 = local write "Output Other Boolean Array"(w563) -> ()
                                }
                                }
                                }
                                frame True {
                                n447 = flat-sequence {
                                frame #0 {
                                w565 = FALSE ("START X")
                                n448 = local write "Output Iterasyon Successful"(0.0 ("Iterasyon Successful")) -> ()
                                n449 = local write "RESET SENS Y"(TRUE ("START X")) -> ()
                                n450 = local write "reset values"(w565) -> ()
                                n451 = local write "pass hz"(w565) -> ()
                                n452 = local write "RESET SENS X"(w565) -> ()
                                n453 = local write "change switch"(w565) -> ()
                                }
                                frame #1 {
                                n454 = local read "Output Other Boolean Array"() -> (w577:bool[])
                                n455 = Replace Array Subset(array=w577, new element #1=TRUE ("new element/subarray"), index #1=4 ("index"), new element #2=FALSE ("new element/subarray"), index #2=3 ("index"), new element #3=FALSE ("new element/subarray"), index #3=2 ("index"), new element #4=FALSE ("new element/subarray"), index #4=1 ("index"), new element #5=FALSE ("new element/subarray"), index #5=0 ("index")) -> (w578:bool[])
                                n456 = local write "Output Other Boolean Array"(w578) -> ()
                                }
                                }
                                }
                              }
                            }
                            frame True {
                              n457 = local read "Iterasyon Successful"() -> (w580:dbl)
                              n458 = Greater Or Equal?(x=w580, y=4.0) -> (x >= y?=w579:bool)
                              n459 = case shown="True" w579 {
                                frame False {
                                n460 = flat-sequence {
                                frame #0 {
                                w585 = FALSE ("START X")
                                n461 = local read "denge degeri"() -> (w584:dbl)
                                n462 = case shown="5" w584 {
                                frame 1 {
                                n463 = local write "Denge Seçimi"(u32 4 ("Çalıştırmak istediğiniz Programı Seçin")) -> ()
                                }
                                frame 2 {
                                n464 = local write "Denge Seçimi"(u32 3 ("Çalıştırmak istediğiniz Programı Seçin")) -> ()
                                }
                                frame 3 {
                                n465 = local write "Denge Seçimi"(u32 5 ("Çalıştırmak istediğiniz Programı Seçin")) -> ()
                                }
                                frame 4, Default {
                                n466 = local write "Denge Seçimi"(u32 2 ("Çalıştırmak istediğiniz Programı Seçin")) -> ()
                                }
                                frame 5 {
                                n467 = local write "Denge Seçimi"(u32 1 ("Çalıştırmak istediğiniz Programı Seçin")) -> ()
                                }
                                }
                                n468 = local read "Iterasyon Successful"() -> (w583:dbl)
                                n469 = local write "RESET SENS X"(w585) -> ()
                                n470 = local write "pass hz"(w585) -> ()
                                n471 = local write "RESET SENS Y"(w585) -> ()
                                n472 = local write "reset values"(w585) -> ()
                                n473 = Increment(x=w583) -> (x+1=w582:dbl)
                                n474 = local write "Output Iterasyon Successful"(w582) -> ()
                                n475 = local write "change switch"(TRUE ("kelvin switch")) -> ()
                                }
                                frame #1 {
                                n476 = local read "Output Other Boolean Array"() -> (w602:bool[])
                                n477 = Replace Array Subset(array=w602, new element #1=FALSE ("new element/subarray"), index #1=4 ("index"), new element #2=FALSE ("new element/subarray"), index #2=3 ("index"), new element #3=FALSE ("new element/subarray"), index #3=2 ("index"), new element #4=TRUE ("new element/subarray"), index #4=1 ("index"), new element #5=FALSE ("new element/subarray"), index #5=0 ("index")) -> (w603:bool[])
                                n478 = local write "Output Other Boolean Array"(w603) -> ()
                                }
                                }
                                }
                                frame True {
                                n479 = flat-sequence {
                                frame #0 {
                                n480 = Get Date/Time In Seconds() -> (seconds since 1Jan1904=w605:timestamp)
                                n481 = Get Date/Time String(seconds (now)=w605, want seconds? (F)=TRUE) -> (time string=w604:string)  [unwired: 1 in, 1 out]
                                n482 = local write "end time"(w604) -> ()
                                }
                                frame #1 {
                                n483 = local read "frekans index"() -> (w619:dbl)
                                n484 = local read "set"() -> (w616:u16)
                                n485 = local read "ölçüm"() -> (w623:u16)
                                n486 = local read "control hz array"() -> (w608:dbl[][])
                                n487 = local read "frekans index"() -> (w620:dbl)
                                n488 = local read "control hz array"() -> (w607:dbl[][])
                                n489 = Decrement(x=w616) -> (x-1=w618:u16)
                                n490 = Decrement(x=w623) -> (x-1=w621:u16)
                                n491 = call "change2d.vi"("reset(default false)"=FALSE, "index (col)"=w619, "index (row)"=2, "read/write(T/F)"=TRUE, "2D Array"=w608) -> ("result count"=w617:dbl)  [unwired: 5 in, 1 out]
                                n492 = call "change2d.vi"("reset(default false)"=FALSE, "index (col)"=w620, "index (row)"=1, "read/write(T/F)"=TRUE, "2D Array"=w607) -> ("result count"=w622:dbl)  [unwired: 5 in, 1 out]
                                n493 = Greater Or Equal?(x=w617, y=w618) -> (x >= y?=w613:bool)
                                n494 = Greater Or Equal?(x=w622, y=w621) -> (x >= y?=w612:bool)
                                n495 = And(x=w612, y=w613) -> (x .and. y?=w611:bool)
                                n496 = case shown="True" w611 {
                                frame False {
                                n497 = flat-sequence {
                                frame #0 {
                                n498 = Wait (ms)(milliseconds to wait=u32 500) -> ()  [unwired: 1 out]
                                "continue object" <- TRUE
                                }
                                frame #1 {
                                n499 = local read "ölçüm"() -> (w631:u16)
                                n500 = local read "set"() -> (w632:u16)
                                n501 = Multiply(x=w631, y=w632) -> (x*y=w633:u16)
                                n502 = Multiply(x=u16 2, y=w633) -> (x*y=w629:u16)
                                n503 = local read "extra default values"() -> (w628:dbl[][])
                                n504 = for {
                                N: w629 -> [_]
                                tunnel: w628 -> [w634]
                                i -> [w637]
                                n505 = local read "continue object"() -> (w635:bool)
                                n506 = Quotient & Remainder(x=w637, y=2) -> (x-y*floor(x/y)=w639:i32)  [unwired: 1 out]
                                n507 = Not Equal?(x=w639, y=0) -> (x != y?=w636:bool)
                                n508 = case shown="True" w636 {
                                tunnel: w637 -> [_ w643]
                                tunnel: w635 -> [_ w642]
                                tunnel: w634 -> [_ w641]
                                frame False {
                                }
                                frame True {
                                n509 = case shown="True" w642 {
                                tunnel: w643 -> [_ w645]
                                tunnel: w641 -> [_ w644]
                                frame False {
                                }
                                frame True {
                                n510 = local read "frekans index"() -> (w646:dbl)
                                n511 = Index Array(array=w644, index (row)=w646, index (col)=w645) -> (element=w648:dbl)
                                n512 = Equal?(x=w648, y=0.0) -> (x = y?=w647:bool)
                                n513 = case shown="True" w647 {
                                tunnel: w646 -> [_ w660]
                                tunnel: w644 -> [_ w659]
                                tunnel: w645 -> [_ w658]
                                frame False {
                                }
                                frame True {
                                n514 = local read "input values"() -> (w651:dbl[])
                                n515 = Decrement(x=w658) -> (x-1=w657:i32)
                                n516 = Index Array(array=w651, index #1=19 ("index"), index #2=9 ("index")) -> (element #1=w653:dbl, element #2=w652:dbl)
                                n517 = Replace Array Subset(array=w659, new element #1=w652, index (row) #1=w660, index (col) #1=w657, new element #2=w653, index (row) #2=w660, index (col) #2=w658) -> (w650:dbl[][])
                                n518 = local write "extra default values"(w650) -> ()
                                n519 = local write "continue object"(FALSE ("continue object")) -> ()
                                }
                                }
                                }
                                }
                                }
                                }
                                }
                                }
                                frame #2 {
                                n520 = Wait (ms)(milliseconds to wait=u32 500) -> ()  [unwired: 1 out]
                                }
                                frame #3 {
                                n521 = flat-sequence {
                                frame #0 {
                                n522 = local read "input values"() -> (w666:dbl[])
                                n523 = Array Subset(array=w666, index=9, length=20) -> (w663:dbl[])
                                n524 = Array To Cluster(array=w663) -> (cluster=w662:T5)
                                n525 = local read "default values"() -> (w669:T3)
                                n526 = local read "frekans index"() -> (w667:dbl)
                                n527 = Replace Array Subset(array=w669, new element=w662, index=w667) -> (w668:T3)
                                n528 = local write "default values"(w668) -> ()
                                }
                                frame #1 {
                                n529 = local read "frekans index"() -> (w673:dbl)
                                n530 = local read "control hz array"() -> (w670:dbl[][])
                                n531 = call "change2d.vi"("reset(default false)"=FALSE, "index (col)"=w673, "index (row)"=1, "read/write(T/F)"=FALSE, "2D Array"=w670) -> ("2D Array Result"=w671:dbl[][])  [unwired: 5 in, 1 out]
                                n532 = local write "control hz array"(w671) -> ()
                                }
                                }
                                }
                                frame #4 {
                                w676 = FALSE ("START X")
                                n533 = local write "RESET SENS X"(w676) -> ()
                                n534 = local write "pass hz"(w676) -> ()
                                n535 = local write "RESET SENS Y"(w676) -> ()
                                n536 = local write "change switch"(w676) -> ()
                                n537 = local write "reset values"(TRUE ("reset values")) -> ()
                                }
                                frame #5 {
                                n538 = local read "Output Other Boolean Array"() -> (w688:bool[])
                                n539 = Replace Array Subset(array=w688, new element #1=FALSE ("new element/subarray"), index #1=4 ("index"), new element #2=FALSE ("new element/subarray"), index #2=3 ("index"), new element #3=TRUE ("new element/subarray"), index #3=2 ("index"), new element #4=FALSE ("new element/subarray"), index #4=1 ("index"), new element #5=FALSE ("new element/subarray"), index #5=0 ("index")) -> (w689:bool[])
                                n540 = local write "Output Other Boolean Array"(w689) -> ()
                                }
                                }
                                }
                                frame True {
                                n541 = flat-sequence {
                                frame #0 {
                                n542 = local write "continue object"(TRUE ("continue object")) -> ()
                                n543 = Wait (ms)(milliseconds to wait=u32 500) -> ()  [unwired: 1 out]
                                }
                                frame #1 {
                                n544 = local read "ölçüm"() -> (w695:u16)
                                n545 = local read "set"() -> (w696:u16)
                                n546 = Multiply(x=w695, y=w696) -> (x*y=w697:u16)
                                n547 = Multiply(x=u16 2, y=w697) -> (x*y=w693:u16)
                                n548 = local read "extra default values"() -> (w692:dbl[][])
                                n549 = for {
                                N: w693 -> [_]
                                tunnel: w692 -> [w698]
                                i -> [w701]
                                n550 = local read "continue object"() -> (w699:bool)
                                n551 = Quotient & Remainder(x=w701, y=2) -> (x-y*floor(x/y)=w703:i32)  [unwired: 1 out]
                                n552 = Not Equal?(x=w703, y=0) -> (x != y?=w700:bool)
                                n553 = case shown="True" w700 {
                                tunnel: w701 -> [_ w707]
                                tunnel: w699 -> [_ w706]
                                tunnel: w698 -> [_ w705]
                                frame False {
                                }
                                frame True {
                                n554 = case shown="True" w706 {
                                tunnel: w707 -> [_ w709]
                                tunnel: w705 -> [_ w708]
                                frame False {
                                }
                                frame True {
                                n555 = local read "frekans index"() -> (w710:dbl)
                                n556 = Index Array(array=w708, index (row)=w710, index (col)=w709) -> (element=w712:dbl)
                                n557 = Equal?(x=w712, y=0.0) -> (x = y?=w711:bool)
                                n558 = case shown="True" w711 {
                                tunnel: w710 -> [_ w724]
                                tunnel: w708 -> [_ w723]
                                tunnel: w709 -> [_ w722]
                                frame False {
                                }
                                frame True {
                                n559 = local read "input values"() -> (w715:dbl[])
                                n560 = Decrement(x=w722) -> (x-1=w721:i32)
                                n561 = Index Array(array=w715, index #1=19 ("index"), index #2=9 ("index")) -> (element #1=w717:dbl, element #2=w716:dbl)
                                n562 = Replace Array Subset(array=w723, new element #1=w716, index (row) #1=w724, index (col) #1=w721, new element #2=w717, index (row) #2=w724, index (col) #2=w722) -> (w714:dbl[][])
                                n563 = local write "extra default values"(w714) -> ()
                                n564 = local write "continue object"(FALSE ("continue object")) -> ()
                                }
                                }
                                }
                                }
                                }
                                }
                                }
                                }
                                frame #2 {
                                n565 = Wait (ms)(milliseconds to wait=u32 500) -> ()  [unwired: 1 out]
                                }
                                frame #3 {
                                n566 = flat-sequence {
                                frame #0 {
                                n567 = local read "ölçüm"() -> (w733:u16)
                                n568 = local read "input values"() -> (w726:dbl[])
                                n569 = local read "extra default values"() -> (w730:dbl[][])
                                n570 = local read "set"() -> (w734:u16)
                                n571 = Multiply(x=w733, y=w734) -> (x*y=w735:u16)
                                n572 = Multiply(x=u16 2, y=w735) -> (x*y=w731:u16)
                                n573 = for {
                                N: w731 -> [_]
                                tunnel: w730 -> [w740]
                                tunnel: [w739] -> w729 mode=indexing
                                i -> [w741]
                                n574 = local read "frekans index"() -> (w737:dbl)
                                n575 = Index Array(array=w740, index (row)=w737, index (col)=w741) -> (element=w739:dbl)
                                n576 = Wait (ms)(milliseconds to wait=u32 50) -> ()  [unwired: 1 out]
                                }
                                n577 = Insert Into Array(array=w726, index=51, new element=w729) -> (w728:dbl[])
                                n578 = local read "Sheet name"() -> (w727:string)
                                n579 = call "excel.vi"("1d array"=w728, "Sheet name"=w727) -> ()  [unwired: 9 in]
                                }
                                frame #1 {
                                n580 = local read "frekans index"() -> (w744:dbl)
                                n581 = local read "control hz array"() -> (w746:dbl[][])
                                n582 = call "change2d.vi"("reset(default false)"=FALSE, "index (col)"=w744, "index (row)"=1, "read/write(T/F)"=FALSE, "2D Array"=w746) -> ("2D Array Result"=w747:dbl[][])  [unwired: 5 in, 1 out]
                                n583 = local write "control hz array"(w747) -> ()
                                }
                                }
                                }
                                frame #4 {
                                w748 = FALSE ("START X")
                                n584 = local write "RESET SENS X"(w748) -> ()
                                n585 = local write "reset values"(TRUE ("reset values")) -> ()
                                n586 = local write "pass hz"(w748) -> ()
                                n587 = local write "RESET SENS Y"(w748) -> ()
                                n588 = local write "change switch"(w748) -> ()
                                }
                                frame #5 {
                                n589 = local read "Output Other Boolean Array"() -> (w760:bool[])
                                n590 = Replace Array Subset(array=w760, new element #1=FALSE ("new element/subarray"), index #1=4 ("index"), new element #2=FALSE ("new element/subarray"), index #2=3 ("index"), new element #3=TRUE ("new element/subarray"), index #3=2 ("index"), new element #4=FALSE ("new element/subarray"), index #4=1 ("index"), new element #5=FALSE ("new element/subarray"), index #5=0 ("index")) -> (w761:bool[])
                                n591 = local write "Output Other Boolean Array"(w761) -> ()
                                }
                                }
                                }
                                }
                                }
                                }
                                }
                              }
                            }
                          }
                        }
                      }
                    }
                    frame True {
                      n592 = flat-sequence {
                        frame #0 {
                          n593 = local write "reset values"(TRUE ("reset values")) -> ()
                          n594 = local write "pass hz"(TRUE ("pass hz")) -> ()
                        }
                        frame #1 {
                          w764 = FALSE ("pass hz")
                          n595 = local write "RESET SENS X"(w764) -> ()
                          n596 = local write "change switch"(w764) -> ()
                          n597 = local write "RESET SENS Y"(w764) -> ()
                        }
                        frame #2 {
                          n598 = local read "Output Other Boolean Array"() -> (w775:bool[])
                          n599 = Replace Array Subset(array=w775, new element #1=FALSE ("new element/subarray"), index #1=4 ("index"), new element #2=FALSE ("new element/subarray"), index #2=3 ("index"), new element #3=FALSE ("new element/subarray"), index #3=2 ("index"), new element #4=FALSE ("new element/subarray"), index #4=1 ("index"), new element #5=TRUE ("new element/subarray"), index #5=0 ("index")) -> (w776:bool[])
                          n600 = local write "Output Other Boolean Array"(w776) -> ()
                        }
                      }
                    }
                  }
                }
              }
            }
          }
        }
        frame #1 {
          n601 = local read "AD F/P Array"() -> (w781:dbl[][])
          n602 = local read "10R F/P Array"() -> (w780:dbl[][])
          n603 = local read "1R F/P Array"() -> (w779:dbl[][])
          n604 = local read "Wagner F/P Array"() -> (w778:dbl[][])
          n605 = local read "Kelvin F/P Array"() -> (w777:dbl[][])
          n606 = local read "control hz array"() -> (w787:dbl[][])
          n607 = local read "extra default values"() -> (w786:dbl[][])
          n608 = local read "F Values Array"() -> (w788:dbl[][])
          n609 = local read "default values"() -> (w784:T3)
          n610 = local read "F/P Array Cluster"() -> (w783:T1)
          n611 = local read "Cluster"() -> (w789:T2)
          n612 = Bundle By Name(cluster=w783, "AD F/P Array"=w781, "10R F/P Array"=w780, "1R F/P Array"=w779, "Wagner F/P Array"=w778, "Kelvin F/P Array"=w777) -> (w782:T1)
          n613 = Bundle By Name(cluster=w789, "F Values Array"=w788, "control hz array"=w787, "extra default values"=w786) -> (w785:T2)
          n614 = local write "output default values"(w784) -> ()
          n615 = local write "Output F/P Array Cluster"(w782) -> ()
          n616 = local write "Output Cluster"(w785) -> ()
        }
      }
    }
  }
